vi "SDT_ReadFileBlock.vi"(8 "error in":errorcluster, 9 "MeasureInfo":T7[](array[typedef]) {"MeasFCSInfo"."fcs_decay_calc" format="%x"; "MeasStopInfo"."flags" format="x%x"; "MeasureInfo_PartB"."mod_type2" format="%016x"; "MeasureInfo_PartB"."mod_type1" format="%016x"}, 10 "bhfile_header":T6 {"chksum" format="x%x"; "header_valid" format="x%x"}, 11 "SDTFileRefnum":refnum<file>) -> (0 "error out":errorcluster, 1 "DecayMatrix":cluster{"Waveform Graph":sgl[]}[][](array[cluster]), 2 "IntensityImage":cluster{"Intensity Graph":u8[][]}[](array[cluster]), 3 "BHFileBlockHeader_interpreted":T1[](array[typedef]) {"lblock_Contents" items=["DECAY_BLOCK"=0, "PAGE_BLOCK"=16, "FCS_BLOCK"=32, "FIDA_BLOCK"=48, "FILDA_BLOCK"=64, "MCS_BLOCK"=80, "IMG_BLOCK"=96, "MCST_BLOCK"=112, "IMG_MCS_BLOCK"=128, "MOM_BLOCK"=144, "IMG_INT_BLOCK"=160, "IMG_WF_BLOCK"=176, "IMG_LIFE_BLOCK"=192]; "CreationMode" items=["NOT_USED"=0, "MEAS_DATA"=1, "FLOW_DATA"=2, "MEAS_DATA_FROM_FILE"=3, "CALC_DATA"=4, "SIM_DATA"=5, "FIFO_DATA"=8, "FIFO_DATA_FROM_FILE"=9, "MOM_DATA"=10, "MOM_DATA_FROM_FILE"=11]; "Contents" items=["DECAY_BLOCK"=0, "PAGE_BLOCK"=16, "FCS_BLOCK"=32, "FIDA_BLOCK"=48, "FILDA_BLOCK"=64, "MCS_BLOCK"=80, "IMG_BLOCK"=96, "MCST_BLOCK"=112, "IMG_MCS_BLOCK"=128, "MOM_BLOCK"=144, "IMG_INT_BLOCK"=160, "IMG_WF_BLOCK"=176, "IMG_LIFE_BLOCK"=192]; "DataType" items=["DATA_USHORT (U16)"=0, "DATA_ULONG (U32)"=256, "DATA_DBL (DBL64)"=512]; "BHFileBlockHeader"."lblock_no" format="x%x"; "BHFileBlockHeader"."block_type" format="%x"}, 4 "FCS_Block":cluster{"XY Graph":cluster{dbl[], dbl[]}}[](array[cluster]), 5 "SumOfDecays":dbl[][](graph))   [LabVIEW 2019]
doc: "This VI is a SubVI to SDT_ReadFile.vi. It reads the BHFileBlockHeader and data blocks in a SDT-file from disc.\nFor a description of the *.sdt file format see: SPC_data_file_structure.h\n\ninfo@becker-hickl.com"
uses:
  SPC_Controls/MeasureInfo.ctl
  SPC_Controls/MeasureInfo_PartB.ctl
  SPC_Controls/MeasStopInfo.ctl
  SPC_Controls/MeasFCSInfo.ctl
  SPC_Controls/MeasureInfo_PartE.ctl
  SPC_Controls/MeasHISTInfo.ctl
  SPC_Controls/HISTInfoExt.ctl
  SPC_Controls/MeasureInfo_PartI.ctl
  SPC_Controls/MeasureInfo_PartK.ctl
  SPC_Controls/MeasureInfo_PartM.ctl
  SPC_Controls/bhfile_header.ctl
  SPC_Controls/BHFileBlockHeader_interpreted.ctl
  SPC_Controls/BHFileBlockHeader.ctl
  SPC_Controls/BlockType_DataType.ctl
  SPC_Controls/BlockType_Contents.ctl
  SPC_Controls/BlockType_CreationMode.ctl
panel:
  # "block_type"
  # "lblock_no"
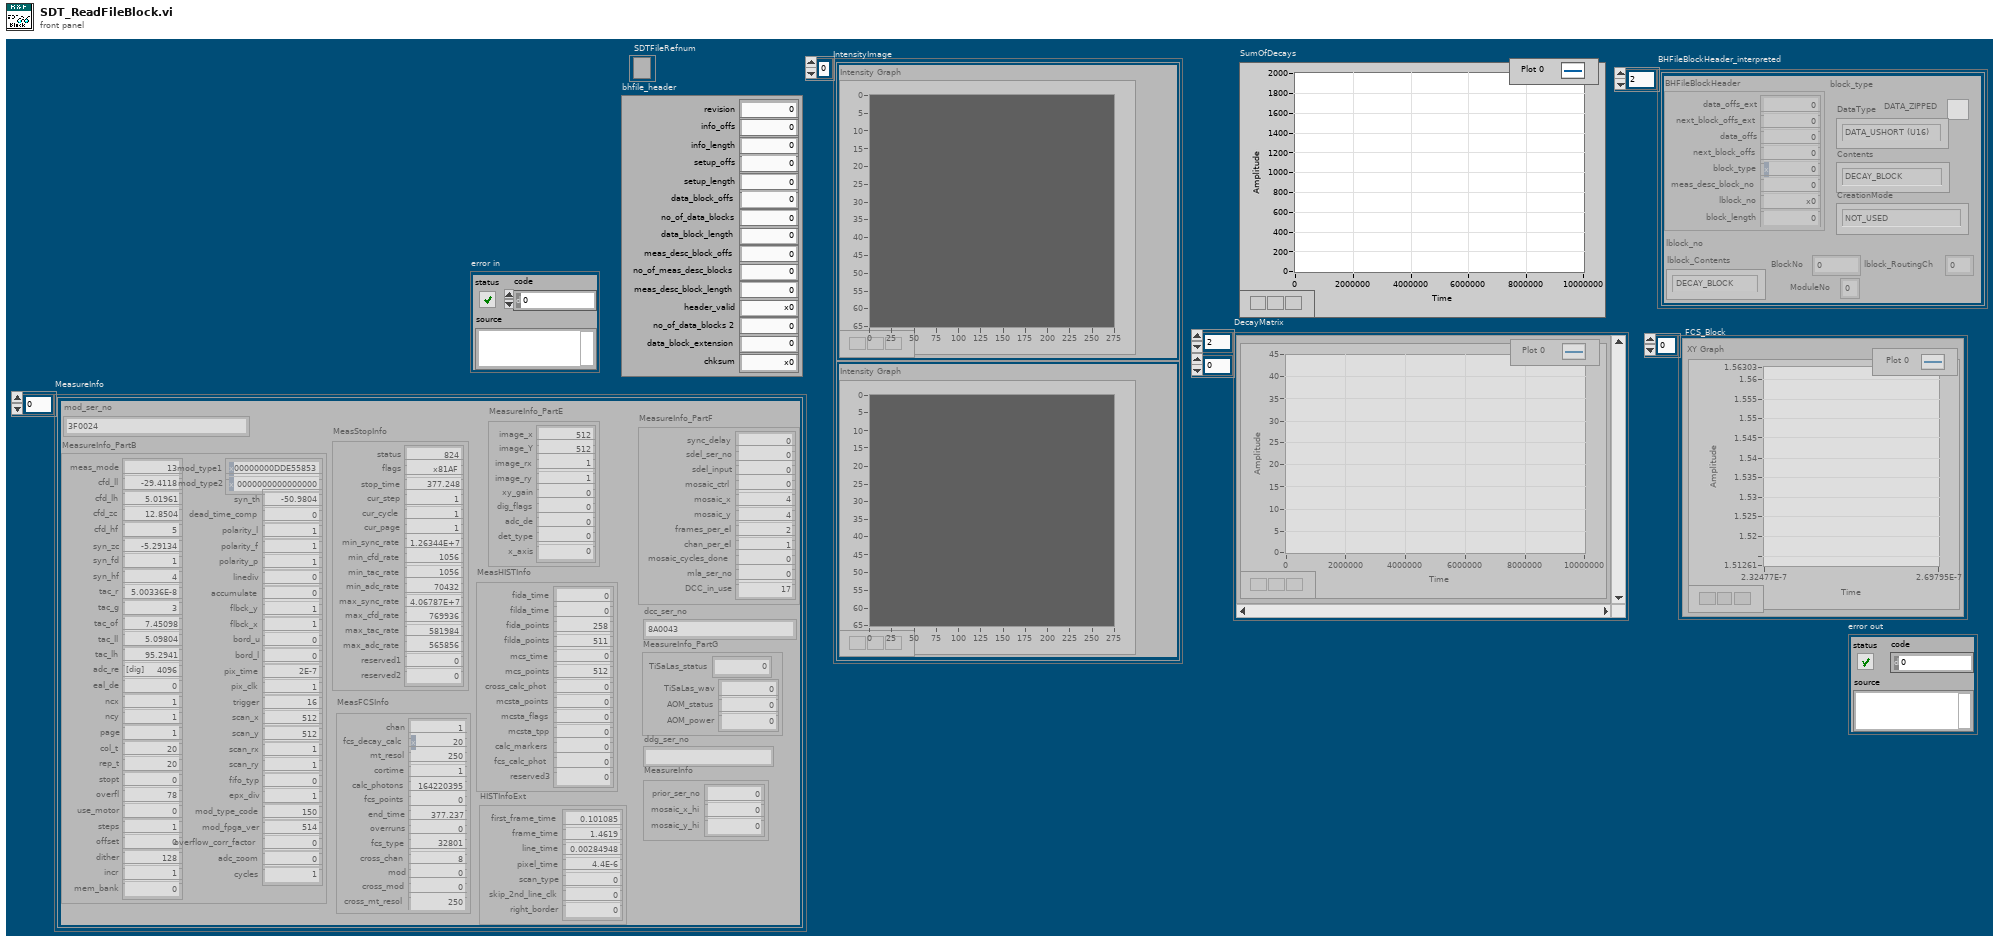
[diagram p1: front panel]
types:
  T1 = typedef "BHFileBlockHeader_interpreted.ctl" = cluster{"BHFileBlockHeader":T2, "DATA_ZIPPED":bool, "DataType":T3, "Contents":T4, "CreationMode":T5, "lblock_Contents":T4, "ModuleNo":u8, "BlockNo":u32, "lblock_RoutingCh":u32}
  T2 = typedef "BHFileBlockHeader.ctl" = cluster{"data_offs_ext":u8, "next_block_offs_ext":u8, "data_offs":u32, "next_block_offs":u32, "block_type":u16, "meas_desc_block_no":i16, "lblock_no":u32, "block_length":u32}
  T3 = typedef "BlockType_DataType.ctl" = u16
  T4 = typedef "BlockType_Contents.ctl" = u16
  T5 = typedef "BlockType_CreationMode.ctl" = u16
  T6 = typedef "bhfile_header.ctl" = cluster{"revision":i16, "info_offs":i32, "info_length":i16, "setup_offs":i32, "setup_length":u16, "data_block_offs":i32, "no_of_data_blocks":i16, "data_block_length":u32, "meas_desc_block_offs":i32, "no_of_meas_desc_blocks":i16, "meas_desc_block_length":i16, "header_valid":u16, "no_of_data_blocks 2":u32, "data_block_extension":u16, "chksum":u16}
  T7 = typedef "MeasureInfo.ctl" = cluster{"mod_ser_no":string, "MeasureInfo_PartB":T8, "MeasStopInfo":T9, "MeasFCSInfo":T10, "MeasureInfo_PartE":T11, "MeasHISTInfo":T12, "HISTInfoExt":T13, "MeasureInfo_PartF":T14, "dcc_ser_no":string, "MeasureInfo_PartG":T15, "ddg_ser_no":string, "MeasureInfo":T16}
  T8 = typedef "MeasureInfo_PartB.ctl" = cluster{"meas_mode":i16, "cfd_ll":sgl, "cfd_lh":sgl, "cfd_zc":sgl, "cfd_hf":sgl, "syn_zc":sgl, "syn_fd":i16, "syn_hf":sgl, "tac_r":sgl, "tac_g":i16, "tac_of":sgl, "tac_ll":sgl, "tac_lh":sgl, "adc_re":i16, "eal_de":i16, "ncx":i16, "ncy":i16, "page":u16, "col_t":sgl, "rep_t":sgl, "stopt":i16, "overfl":i8, "use_motor":i16, "steps":u16, "offset":sgl, "dither":i16, "incr":i16, "mem_bank":i16, "mod_type1":u64, "mod_type2":u64, "syn_th":sgl, "dead_time_comp":i16, "polarity_l":i16, "polarity_f":i16, "polarity_p":i16, "linediv":i16, "accumulate":i16, "flbck_y":i32, "flbck_x":i32, "bord_u":i32, "bord_l":i32, "pix_time":sgl, "pix_clk":i16, "trigger":i16, "scan_x":i32, "scan_y":i32, "scan_rx":i32, "scan_ry":i32, "fifo_typ":i16, "epx_div":i32, "mod_type_code":u16, "mod_fpga_ver":u16, "overflow_corr_factor":sgl, "adc_zoom":i32, "cycles":i32}
  T9 = typedef "MeasStopInfo.ctl" = cluster{"status":u16, "flags":u16, "stop_time":sgl, "cur_step":i32, "cur_cycle":i32, "cur_page":i32, "min_sync_rate":sgl, "min_cfd_rate":sgl, "min_tac_rate":sgl, "min_adc_rate":sgl, "max_sync_rate":sgl, "max_cfd_rate":sgl, "max_tac_rate":sgl, "max_adc_rate":sgl, "reserved1":i32, "reserved2":sgl}
  T10 = typedef "MeasFCSInfo.ctl" = cluster{"chan":u16, "fcs_decay_calc":u16, "mt_resol":u32, "cortime":sgl, "calc_photons":u32, "fcs_points":i32, "end_time":sgl, "overruns":u16, "fcs_type":u16, "cross_chan":u16, "mod":u16, "cross_mod":u16, "cross_mt_resol":u32}
  T11 = typedef "MeasureInfo_PartE.ctl" = cluster{"image_x":i32, "image_Y":i32, "image_rx":i32, "image_ry":i32, "xy_gain":i16, "dig_flags":i16, "adc_de":i16, "det_type":i16, "x_axis":i16}
  T12 = typedef "MeasHISTInfo.ctl" = cluster{"fida_time":sgl, "filda_time":sgl, "fida_points":i32, "filda_points":i32, "mcs_time":sgl, "mcs_points":i32, "cross_calc_phot":u32, "mcsta_points":u16, "mcsta_flags":u16, "mcsta_tpp":u32, "calc_markers":u32, "fcs_calc_phot":u32, "reserved3":u32}
  T13 = typedef "HISTInfoExt.ctl" = cluster{"first_frame_time":sgl, "frame_time":sgl, "line_time":sgl, "pixel_time":sgl, "scan_type":i16, "skip_2nd_line_clk":i16, "right_border":u32}
  T14 = typedef "MeasureInfo_PartI.ctl" = cluster{"sync_delay":sgl, "sdel_ser_no":u16, "sdel_input":i8, "mosaic_ctrl":i8, "mosaic_x":u8, "mosaic_y":u8, "frames_per_el":i16, "chan_per_el":i16, "mosaic_cycles_done":i32, "mla_ser_no":u16, "DCC_in_use":u8}
  T15 = typedef "MeasureInfo_PartK.ctl" = cluster{"TiSaLas_status":u16, "TiSaLas_wav":u16, "AOM_status":u8, "AOM_power":u8}
  T16 = typedef "MeasureInfo_PartM.ctl" = cluster{"prior_ser_no":i32, "mosaic_x_hi":u8, "mosaic_y_hi":u8}
  T17 = enum16{"big-endian, network order", "native, host order", "little-endian"}
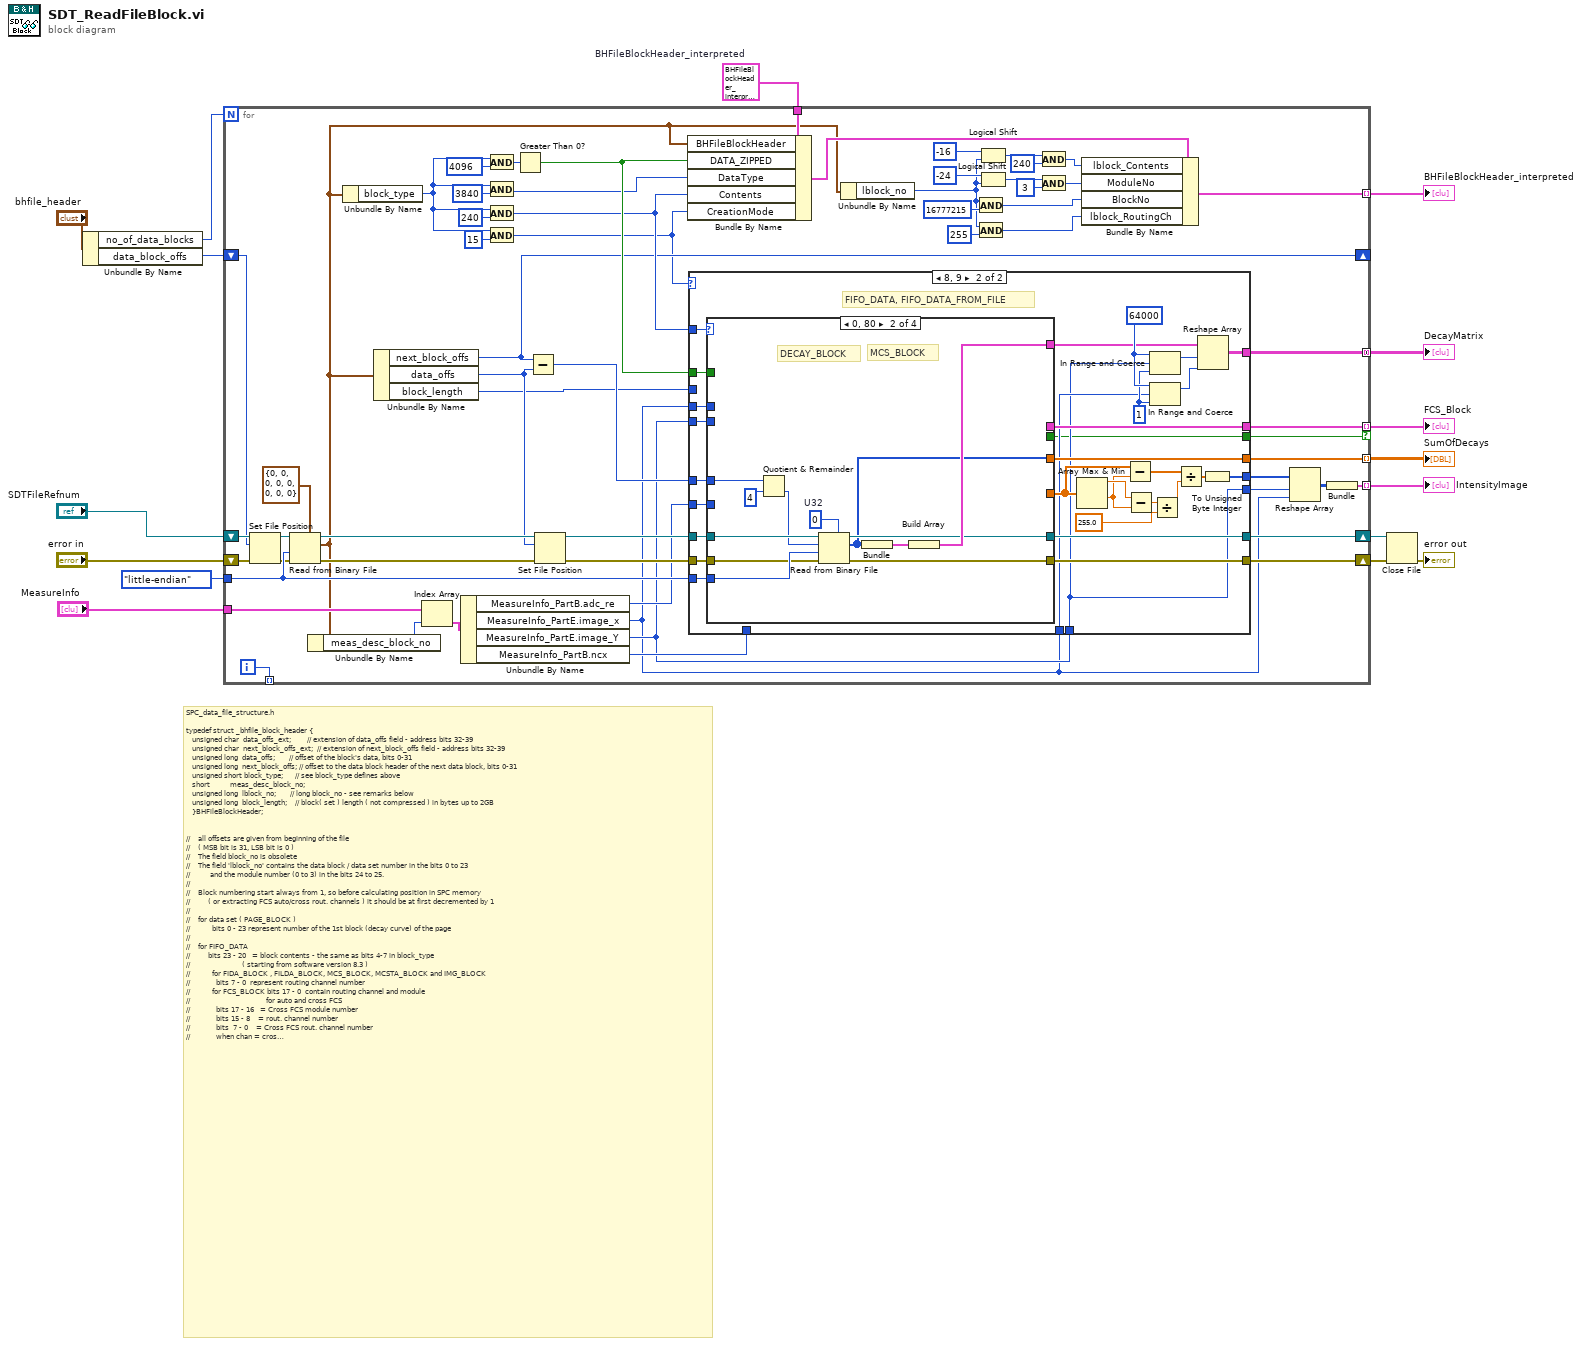
[diagram p0: block diagram]
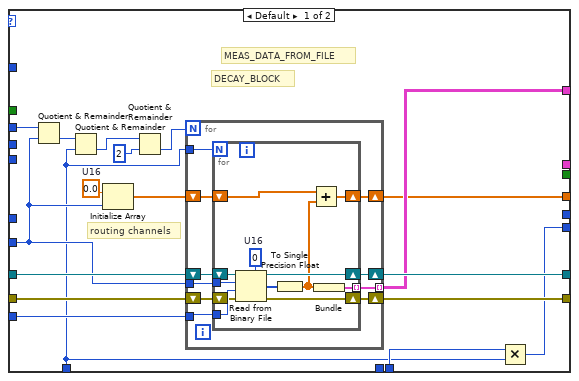
[diagram p2: hidden frame]
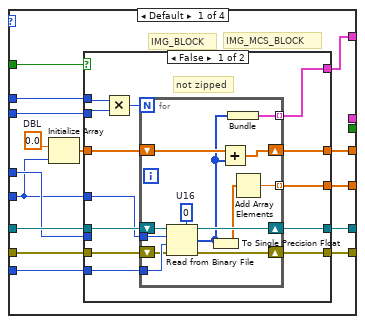
[diagram p3: hidden frame]
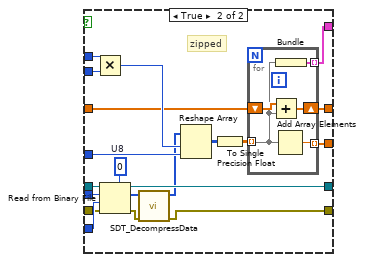
[diagram p4: hidden frame]
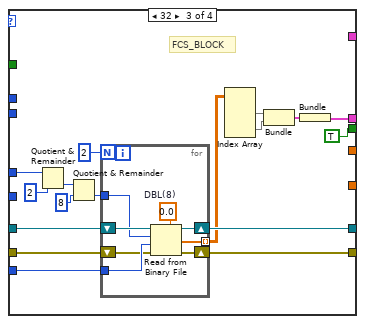
[diagram p5: hidden frame]
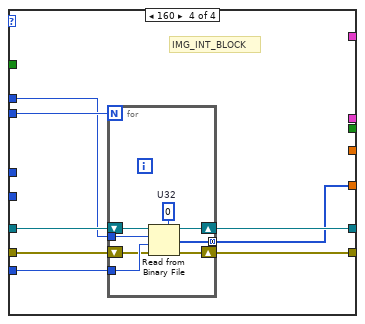
[diagram p6: hidden frame]
diagram:
  w3 = T1 {"BHFileBlockHeader"={"data_offs_ext"=0, "next_block_offs_ext"=0, "data_offs"=0, "next_block_offs"=0, "block_type"=0, "meas_desc_block_no"=0, "lblock_no"=0, "block_length"=0}, "DATA_ZIPPED"=FALSE, "DataType"=0, "Contents"=0, "CreationMode"=11, "lblock_Contents"=128, "ModuleNo"=0, "BlockNo"=0, "lblock_RoutingCh"=0}  # BHFileBlockHeader_interpreted
  # "SPC_data_file_structure.h\n\ntypedef struct _bhfile_block_header {\n   unsigned char  data_offs_ext;        // extension of data_offs field - address bits 32-39\n   unsigned char  next_block_offs_ext;  // extension of next_block_offs field - address bits 32-39\n   unsigned long  data_offs;       // offset of the block's data, bits 0-31  \n   unsigned long  next_block_offs; // offset to the data block header of the next data block, bits 0-31 \n   unsigned short block_type;      // see block_type defines above\n   short          meas_desc_block_no;\n   unsigned long  lblock_no;       // long block_no - see remarks below\n   unsigned long  block_length;    // block( set ) length ( not compressed ) in bytes up to 2GB\n   }BHFileBlockHeader;\n\n\n//    all offsets are given from beginning of the file\n//    ( MSB bit is 31, LSB bit is 0 )\n//    The field block_no is obsolete\n//    The field 'lblock_no' contains the data block / data set number in the bits 0 to 23 \n//          and the module number (0 to 3) in the bits 24 to 25.\n//\n//    Block numbering start always from 1, so before calculating position in SPC memory \n//         ( or extracting FCS auto/cross rout. channels ) it should be at first decremented by 1\n//    \n//    for data set ( PAGE_BLOCK ) \n//           bits 0 - 23 represent number of the 1st block (decay curve) of the page\n//\n//    for FIFO_DATA \n//         bits 23 - 20   = block contents - the same as bits 4-7 in block_type\n//                          ( starting from software version 8.3 )\n//           for FIDA_BLOCK , FILDA_BLOCK, MCS_BLOCK, MCSTA_BLOCK and IMG_BLOCK\n//             bits 7 - 0  represent routing channel number\n//           for FCS_BLOCK bits 17 - 0  contain routing channel and module \n//                                      for auto and cross FCS\n//             bits 17 - 16   = Cross FCS module number\n//             bits 15 - 8    = rout. channel number   \n//             bits  7 - 0    = Cross FCS rout. channel number   \n//             when chan = cross_chan and mod == cross_mod - Auto FCS, \n//                           otherwise - Cross FCS\n//    for MOM_DATA \n//         bits 23 - 20   = block(set) contents - the same as bits 4-7 in block_type\n//         bits 19 -  0   = number of the data set\nee"
  n1 = Unbundle By Name("bhfile_header") -> ("no_of_data_blocks"=w11:i16, "data_block_offs"=w12:i32)
  n2 = for {
    N: w11 -> [_]
    tunnel: T17."little-endian" ("byte order (0:big-endian, network order)") -> [w60]
    tunnel: [w61] -> w16 mode=indexing
    shift-right: [w27] -> _
    shift-left: w12 -> [w59]
    shift-right: [w58] -> w15
    shift-left: "SDTFileRefnum" -> [w64]
    tunnel: [w21] -> w14 mode=concatenating
    tunnel: [w56] -> w13 mode=indexing if=w17
    tunnel: [w55] -> _ mode=indexing
    tunnel: "MeasureInfo" -> [w51]
    shift-right: [w45] -> w10
    shift-left: "error in" -> [w49]
    tunnel: w3 -> [w44]
    tunnel: [w33] -> w2 mode=indexing
    tunnel: [w25] -> w1 mode=indexing
    i -> [w55]
    n3 = Set File Position(offset (in bytes) (0)=w59, refnum=w64, error in=w49) -> (refnum out=w62:refnum<file>, error out=w48:errorcluster)  [unwired: 1 in]
    n4 = Read from Binary File(5:T2 {"data_offs_ext"=0, "next_block_offs_ext"=0, "data_offs"=0, "next_block_offs"=0, "block_type"=0, "meas_desc_block_no"=0, "lblock_no"=0, "block_length"=0} ("BHFileBlockHeader"), 8:w48, 9:w60, 11:w62) -> (0:w47:errorcluster, 2:w29:T2, 3:w63:refnum<file>)  [unwired: 2 in, 1 out]
    n5 = Unbundle By Name(w29) -> ("meas_desc_block_no"=w28:i16)
    n6 = Unbundle By Name(w29) -> ("block_type"=w34:u16)
    n7 = Unbundle By Name(w29) -> ("next_block_offs"=w27:u32, "data_offs"=w26:u32, "block_length"=w24:u32)
    n8 = Index Array(array=w51, index=w28) -> (element=w50:T7)
    n9 = Unbundle By Name(w50) -> ("MeasureInfo_PartB.adc_re"=w30:i16, "MeasureInfo_PartE.image_x"=w19:i32, "MeasureInfo_PartE.image_Y"=w22:i32, "MeasureInfo_PartB.ncx"=w23:i16)
    n10 = And(x=w34, y=u16 4096) -> (x .and. y?=w71:u16)
    n11 = And(x=w34, y=u16 3840) -> (x .and. y?=w42:u16)
    n12 = And(x=w34, y=u16 240) -> (x .and. y?=w41:u16)
    n13 = And(x=w34, y=u16 15) -> (x .and. y?=w18:u16)
    n14 = Greater Than 0?(x=w71) -> (x > 0?=w43:bool)
    n15 = Subtract(x=w27, y=w26) -> (x-y=w57:u32)
    n16 = Set File Position(offset (in bytes) (0)=w26, refnum=w63, error in=w47) -> (refnum out=w66:refnum<file>, error out=w46:errorcluster)  [unwired: 1 in]
    n17 = Bundle By Name(cluster=w44, "BHFileBlockHeader"=w29, "DATA_ZIPPED"=w43, "DataType"=w42, "Contents"=w41, "CreationMode"=w18) -> (w39:T1)
    n18 = case shown="8, 9" w18 {
      tunnel: w66 -> [w94 w147]
      tunnel: [w89 w146] -> w25
      tunnel: w43 -> [_ w145]
      tunnel: w60 -> [w93 w144]
      tunnel: [w92 w143] -> w58
      tunnel: w19 -> [_ w142]
      tunnel: w22 -> [_ w141]
      tunnel: w30 -> [w86 w140]
      tunnel: w57 -> [_ w139]
      tunnel: w24 -> [w91 _]
      tunnel: [w90 w120] -> w21
      tunnel: w41 -> [_ w138]
      tunnel: [_ w137] -> w56
      tunnel: w46 -> [w84 w136]
      tunnel: [w83 w135] -> w45
      tunnel: [_ w126] -> w31
      tunnel: w23 -> [w78 _]
      tunnel: [w79 w121] -> w20
      tunnel: w22 -> [w80 w121]
      tunnel: w19 -> [_ w122]
      tunnel: [_ w117] -> w17
      frame Default {
        w87 = sgl 0.0  # U16
        # "routing channels"
        # "MEAS_DATA_FROM_FILE"
        # "DECAY_BLOCK"
        n19 = Quotient & Remainder(x=w91, y=w86) -> (floor(x/y)=w82:u32)  [unwired: 1 out]
        n20 = Quotient & Remainder(x=w82, y=w78) -> (floor(x/y)=w81:u32)  [unwired: 1 out]
        n21 = Initialize Array(w87, w86) -> (w85:sgl[])
        n22 = Quotient & Remainder(x=w81, y=u32 2) -> (floor(x/y)=w77:u32)  [unwired: 1 out]
        n23 = for {
          N: w77 -> [_]
          tunnel: w93 -> [w103]
          tunnel: [w101] -> w90 mode=indexing
          tunnel: w78 -> [w99]
          tunnel: w86 -> [w98]
          shift-right: [w102] -> w92
          shift-left: w94 -> [w104]
          shift-right: [w95] -> w83
          shift-left: w84 -> [w96]
          shift-right: [w100] -> w89
          shift-left: w85 -> [w97]
          n24 = for {
            N: w99 -> [_]
            tunnel: w103 -> [w115]
            shift-right: [w113] -> w102
            shift-left: w104 -> [w116]
            tunnel: w98 -> [w112]
            tunnel: [w111] -> w101 mode=indexing
            shift-right: [w110] -> w100
            shift-left: w97 -> [w109]
            shift-right: [w107] -> w95
            shift-left: w96 -> [w108]
            w114 = u16 0  # U16
            n25 = Read from Binary File(5:w114, 8:w108, 9:w115, 10:w112, 11:w116) -> (0:w107:errorcluster, 2:w106:u16[], 3:w113:refnum<file>)  [unwired: 1 in, 1 out]
            n26 = To Single Precision Float(number=w106) -> (single precision float=w105:sgl[])
            n27 = Add(x=w109, y=w105) -> (x+y=w110:sgl[])
            n28 = Bundle(w105) -> (w111:cluster{sgl[]})  [unwired: 1 in]
          }
        }
        n29 = Multiply(x=w80, y=w78) -> (x*y=w79:i32)
      }
      frame 8, 9 {
        w124 = 1 ("lower limit")
        w125 = 64000 ("upper limit")
        # "FIFO_DATA, FIFO_DATA_FROM_FILE"
        n30 = case shown="0, 80" w138 {
          tunnel: w147 -> [w162 w225 w242 w258]
          tunnel: [w161 w214 _ _] -> w146
          tunnel: w145 -> [w160 _ _ _]
          tunnel: w144 -> [w159 w224 w241 w257]
          tunnel: [w158 w220 w240 w256] -> w143
          tunnel: w142 -> [w157 _ _ w254]
          tunnel: w141 -> [w156 _ _ w255]
          tunnel: w140 -> [w153 _ _ _]
          tunnel: w139 -> [w155 w218 w239 _]
          tunnel: [w148 w221 _ _] -> w123
          tunnel: [_ _ w227 _] -> w137
          tunnel: w136 -> [w151 w216 w229 w253]
          tunnel: [w150 w215 w228 w252] -> w135
          tunnel: [w149 _ _ w251] -> w127
          tunnel: [_ _ TRUE _] -> w117
          frame Default {
            w154 = 0.0  # DBL
            # "IMG_MCS_BLOCK"
            # "IMG_BLOCK"
            n31 = Initialize Array(w154, w153) -> (w152:dbl[])
            n32 = case shown="False" w160 {
              tunnel: w162 -> [w175 w208]
              tunnel: [w174 w200] -> w149
              tunnel: [w172 w207] -> w158
              tunnel: [w167 w201] -> w161
              tunnel: w159 -> [w171 w194]
              tunnel: w157 -> [w169 w206]
              tunnel: w156 -> [w168 w205]
              tunnel: w153 -> [w170 w202]
              tunnel: w155 -> [_ w198]
              tunnel: w152 -> [w166 w193]
              tunnel: w151 -> [w165 w192]
              tunnel: [w164 w190] -> w150
              tunnel: [w163 w189] -> w148
              frame False {
                # "not zipped"
                n33 = Multiply(x=w169, y=w168) -> (x*y=w173:i32)
                n34 = for {
                  N: w173 -> [_]
                  tunnel: w171 -> [w187]
                  shift-right: [w185] -> w172
                  shift-left: w175 -> [w188]
                  tunnel: [w184] -> w174 mode=indexing
                  tunnel: w170 -> [w183]
                  shift-right: [w181] -> w167
                  shift-left: w166 -> [w180]
                  shift-right: [w178] -> w164
                  shift-left: w165 -> [w179]
                  tunnel: [w176] -> w163 mode=indexing
                  w186 = u16 0  # U16
                  n35 = Read from Binary File(5:w186, 8:w179, 9:w187, 10:w183, 11:w188) -> (0:w178:errorcluster, 2:w177:u16[], 3:w185:refnum<file>)  [unwired: 1 in, 1 out]
                  n36 = To Single Precision Float(number=w177) -> (single precision float=w182:sgl[])
                  n37 = Add(x=w180, y=w177) -> (x+y=w181:dbl[])
                  n38 = Bundle(w177) -> (w176:cluster{u16[]})  [unwired: 1 in]
                  n39 = Add Array Elements(numeric array=w182) -> (sum=w184:sgl)
                }
              }
              frame True {
                w195 = u8 0  # U8
                # "zipped"
                n40 = Multiply(x=w206, y=w205) -> (x*y=w203:i32)
                n41 = Read from Binary File(5:w195, 8:w192, 9:w194, 10:w198, 11:w208) -> (0:w191:errorcluster, 2:w199:u8[], 3:w207:refnum<file>)  [unwired: 1 in, 1 out]
                n42 = call "SDT_DecompressData.vi"("ErrorIn"=w191, "CompressedData"=w199) -> ("ErrorOut"=w190:errorcluster, "DecompressedData(U16)"=w196:u16[])  [unwired: 8 in]
                n43 = Reshape Array(w196, w203, w202) -> (w204:u16[][])
                n44 = To Single Precision Float(number=w204) -> (single precision float=w197:sgl[][])
                n45 = for {
                  tunnel: w197 -> [w210] mode=indexing
                  tunnel: [w213] -> w200 mode=indexing
                  shift-right: [w212] -> w201
                  shift-left: w193 -> [w211]
                  tunnel: [w209] -> w189 mode=indexing
                  n46 = Add(x=w211, y=w210) -> (x+y=w212:dbl[])
                  n47 = Add Array Elements(numeric array=w210) -> (sum=w213:sgl)
                  n48 = Bundle(w210) -> (w209:cluster{sgl[]})  [unwired: 1 in]
                }
              }
            }
          }
          frame 0, 80 {
            w223 = u32 0  # U32
            # "DECAY_BLOCK"
            # "MCS_BLOCK"
            n49 = Quotient & Remainder(x=w218, y=u32 4) -> (floor(x/y)=w219:u32)  [unwired: 1 out]
            n50 = Read from Binary File(5:w223, 8:w216, 9:w224, 10:w219, 11:w225) -> (0:w215:errorcluster, 2:w214:u32[], 3:w220:refnum<file>)  [unwired: 1 in, 1 out]
            n51 = Bundle(w214) -> (w222:cluster{u32[]})  [unwired: 1 in]
            n52 = Build Array(w222) -> (w221:cluster{u32[]}[])
          }
          frame 32 {
            # "FCS_BLOCK"
            n53 = Quotient & Remainder(x=w239, y=u32 2) -> (floor(x/y)=w232:u32)  [unwired: 1 out]
            n54 = Quotient & Remainder(x=w232, y=u32 8) -> (floor(x/y)=w231:u32)  [unwired: 1 out]
            n55 = for {
              N: 2 -> [_]
              tunnel: w241 -> [w249]
              tunnel: w231 -> [w246]
              tunnel: [w245] -> w236 mode=indexing
              shift-right: [w247] -> w240
              shift-left: w242 -> [w250]
              shift-right: [w243] -> w228
              shift-left: w229 -> [w244]
              w248 = 0.0  # DBL(8)
              n56 = Read from Binary File(5:w248, 8:w244, 9:w249, 10:w246, 11:w250) -> (0:w243:errorcluster, 2:w245:dbl[], 3:w247:refnum<file>)  [unwired: 1 in, 1 out]
            }
            n57 = Index Array(array=w236) -> (element #1=w235:dbl[], element #2=w234:dbl[])  [unwired: 4 in]
            n58 = Bundle(w235, w234) -> (w233:cluster{dbl[], dbl[]})  [unwired: 1 in]
            n59 = Bundle(w233) -> (w227:cluster{cluster{dbl[], dbl[]}})  [unwired: 1 in]
          }
          frame 160 {
            # "IMG_INT_BLOCK"
            n60 = for {
              N: w255 -> [_]
              tunnel: w257 -> [w265]
              tunnel: w254 -> [w262]
              tunnel: [w261] -> w251 mode=concatenating
              shift-right: [w263] -> w256
              shift-left: w258 -> [w266]
              shift-right: [w259] -> w252
              shift-left: w253 -> [w260]
              w264 = u32 0  # U32
              n61 = Read from Binary File(5:w264, 8:w260, 9:w265, 10:w262, 11:w266) -> (0:w259:errorcluster, 2:w261:u32[], 3:w263:refnum<file>)  [unwired: 1 in, 1 out]
            }
          }
        }
        n62 = Array Max & Min(array=w127) -> (max value=w134:sgl, min value=w133:sgl)  [unwired: 2 out]
        n63 = Subtract(x=w127, y=w133) -> (x-y=w130:sgl[])
        n64 = Subtract(x=w134, y=w133) -> (x-y=w132:sgl)
        n65 = In Range and Coerce(upper limit=w125, x=w121, lower limit=w124) -> (coerced(x)=w119:i32)  [unwired: 1 out]
        n66 = In Range and Coerce(upper limit=w125, x=w122, lower limit=w124) -> (coerced(x)=w118:i32)  [unwired: 1 out]
        n67 = Divide(x=w132, y=sgl 255.0 ("x")) -> (x/y=w128:sgl)
        n68 = Divide(x=w130, y=w128) -> (x/y=w129:sgl[])
        n69 = Reshape Array(w123, w119, w118) -> (w120:cluster{sgl[]}[][])
        n70 = To Unsigned Byte Integer(number=w129) -> (unsigned 8bit integer=w126:u8[])
      }
    }
    n71 = Unbundle By Name(w29) -> ("lblock_no"=w40:u32)
    n72 = And(x=w40, y=u32 16777215) -> (x .and. y?=w36:u32)
    n73 = And(x=w40, y=u32 255) -> (x .and. y?=w35:u32)
    n74 = Logical Shift(y=i16 -16, x=w40) -> (x << y=w53:u32)
    n75 = Logical Shift(y=i16 -24, x=w40) -> (x << y=w69:u32)
    n76 = And(x=w53, y=i16 240) -> (x .and. y?=w38:u32)
    n77 = And(x=w69, y=i16 3) -> (x .and. y?=w37:u32)
    n78 = Bundle By Name(cluster=w39, "lblock_Contents"=w38, "ModuleNo"=w37, "BlockNo"=w36, "lblock_RoutingCh"=w35) -> (w33:T1)
    n79 = Reshape Array(w31, w20, w19) -> (w65:u8[][])
    n80 = Bundle(w65) -> (w61:cluster{u8[][]})  [unwired: 1 in]
  }
  "DecayMatrix" <- w14
  "FCS_Block" <- w13
  "IntensityImage" <- w16
  "BHFileBlockHeader_interpreted" <- w2
  "SumOfDecays" <- w1
  n81 = Close File(refnum=w15, error in=w10) -> (error out=→"error out":errorcluster)  [unwired: 1 out]
